vi "Reversible Drive Train - Jeter Drive.vi"(9 "Flip":bool, 10 "Number In":dbl) -> (2 "Number Out":dbl)   [LabVIEW 2015]
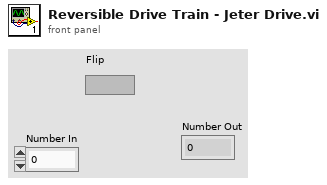
[diagram p1: front panel]
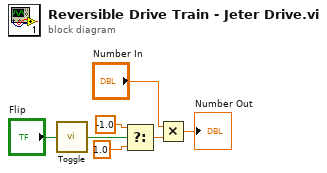
[diagram p0: block diagram]
diagram:
  n1 = call "Toggle.vi"("Input"="Flip") -> ("Output"=w1:bool)
  n2 = Select(t=-1.0, s=w1, f=1.0) -> (s? t:f=w7:dbl)
  n3 = Multiply(x="Number In", y=w7) -> (x*y=→"Number Out":dbl)
